vi "Jan25_prot.vi"() -> ()   [LabVIEW 2020]
uses:
  <vilib>/Utility/error.llb/DialogType.ctl
  <vilib>/Analysis/3filter.llb/Filter Passband Type.ctl
  <vilib>/DAQmx/read.llb/DAQmx Read (Analog 1D DBL NChan 1Samp).vi
  <vilib>/DAQmx/create/channels.llb/DAQmx Create Channel (AI-Voltage-Basic).vi
  <vilib>/DAQmx/configure/timing.llb/DAQmx Timing (Sample Clock).vi
  <vilib>/DAQmx/miscellaneous.llb/DAQmx Fill In Error Info.vi
  <vilib>/Analysis/3filter.llb/Butterworth Filter (DBL).vi
  <vilib>/Utility/file.llb/Write Delimited Spreadsheet (string).vi
  <vilib>/Utility/file.llb/Write Delimited Spreadsheet (DBL).vi
  <vilib>/Analysis/NI_AALBase.lvlib
  <vilib>/ptbypt/NI_PtbyPt.lvlib
panel:
  out "Current value":dbl
  in  "Current sin":bool
  in  "Current":dbl
  in  "Sin f (Hz)":dbl
  out "Delay (sec)":dbl
  out "T tot saved":bool
  out "T start saved":bool
  out "Motor":dynamicdata(graph)
  out "T_next":dbl
  out "T_tot":dbl
  in  "Choose Manual Mode":string(combo)
  out "Actual Swing":bool
  out "N° step Max":i32
  in  "Choose Automatic Mode":string(combo)
  in  "START":bool
  out "Step Number":i32
  out "Step Counted":bool
  out "Time to Peak (sec)":dbl=200.0
  out "Swing ON Time (sec)":dbl
  in  "Only pre-tension load":bool
  out "Gyro":dynamicdata(graph)
  out "Max Square Wave duration (sec)":dbl
  out "Swing Start Time (sec)":dbl
  out "Time Saved":bool
  out "Pre-Tension Load (N)":dbl
  out "Target Load (N)":dbl=2.0
  out "Release":bool
  out "Pull":bool
  in  "Working Mode":string(combo)
  out "Load Cell":dbl
  in  "Pull CMD":bool
  in  "Release CMD":bool
  out "Load Cell":dynamicdata(graph)
  in  "Master Stop":bool
  out "Consumer Loop Speed (ms)":u32
  out "Producer Loop Speed (ms)":u32
  out "Swing":bool
  out "Force Plate":dynamicdata(graph)
  out "Accelerometers":dynamicdata(graph)
  out "Enlapsed Time (sec)":dbl
  # "Choose work mode"
  # "Manual"
  # "Automatic"
  # "Ramp Between-Step Mode"
  # "Ramp Within-Step Mode"
  # "Indicators"
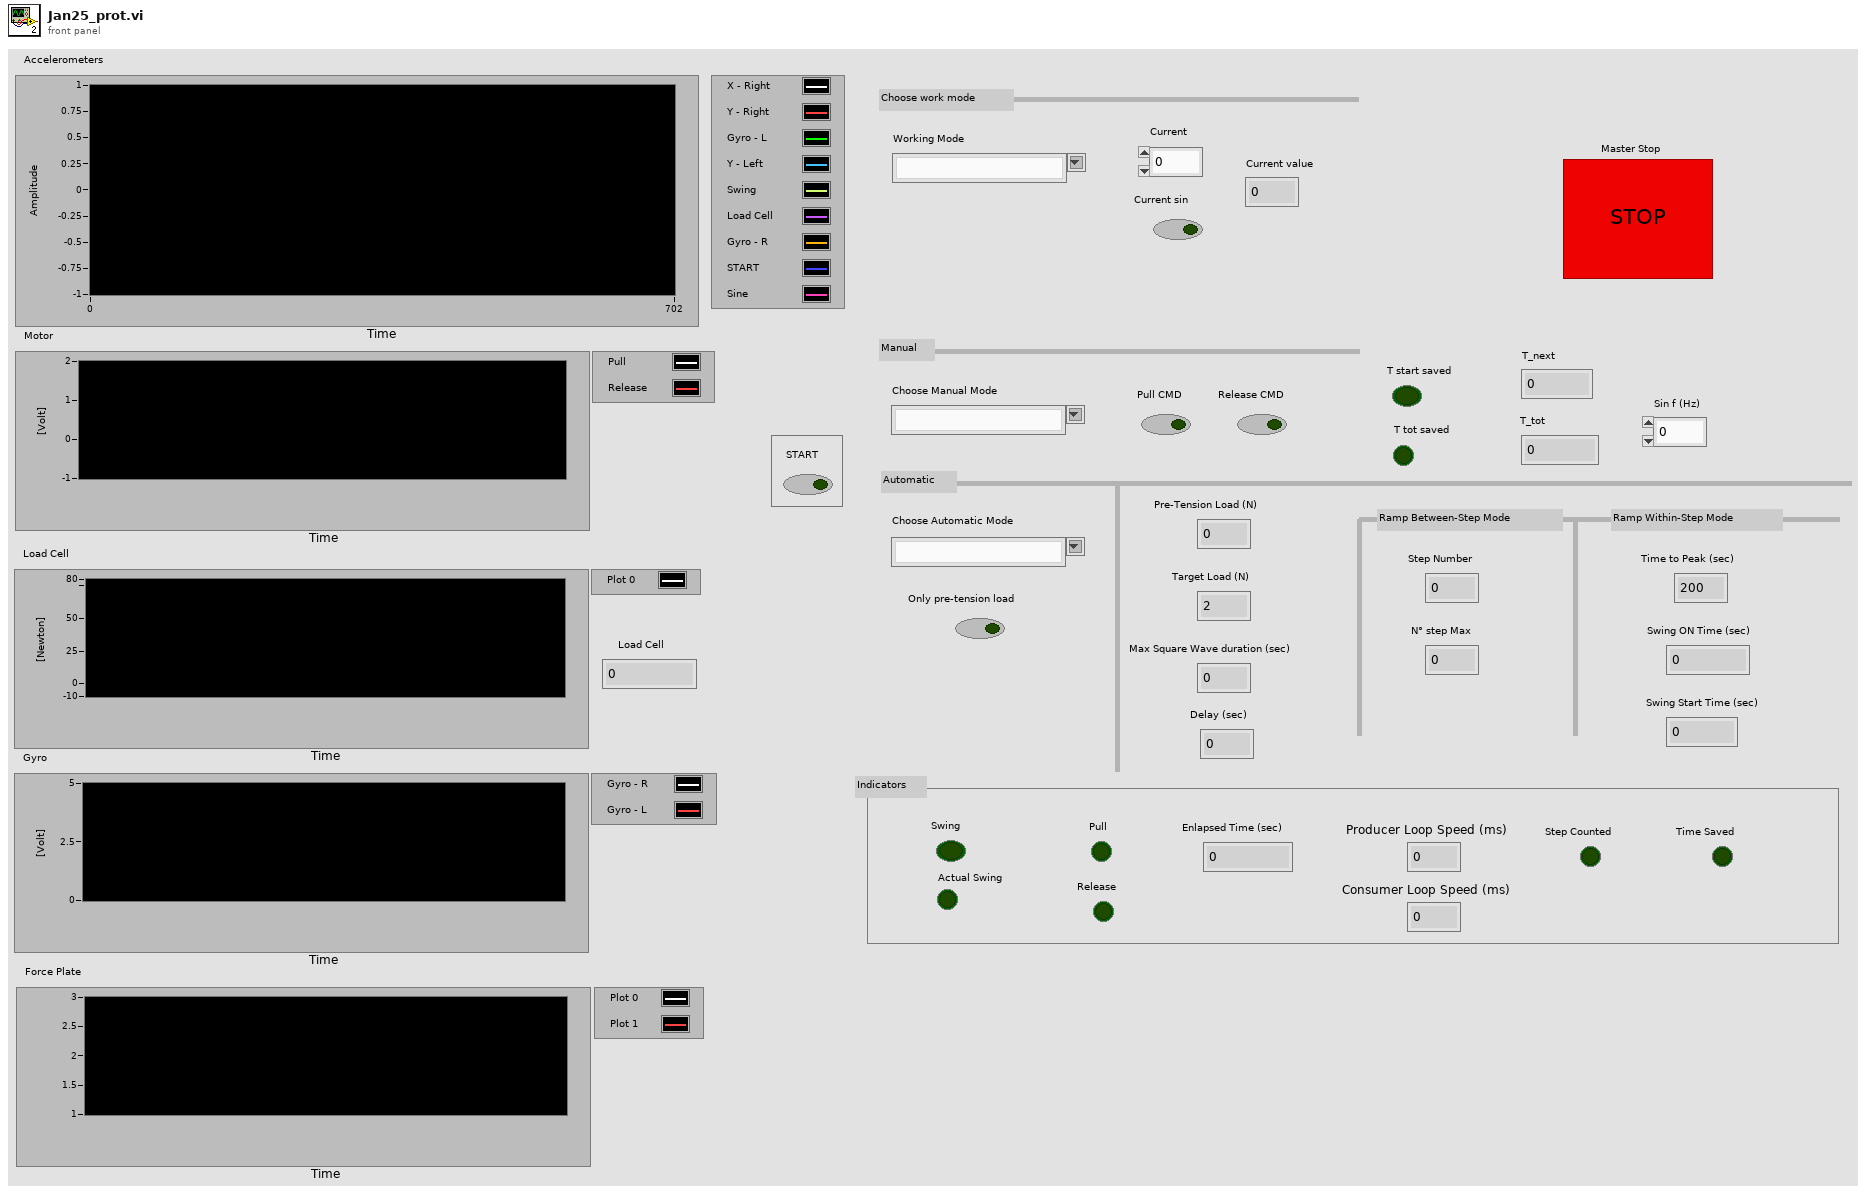
[diagram p1: front panel]
types:
  T1 = typedef "DialogType.ctl" = u16
  T2 = typedef "NI_AALBase.lvlib/Filter Passband Type.ctl" = enum32{"Lowpass", "Highpass", "Bandpass", "Bandstop"}
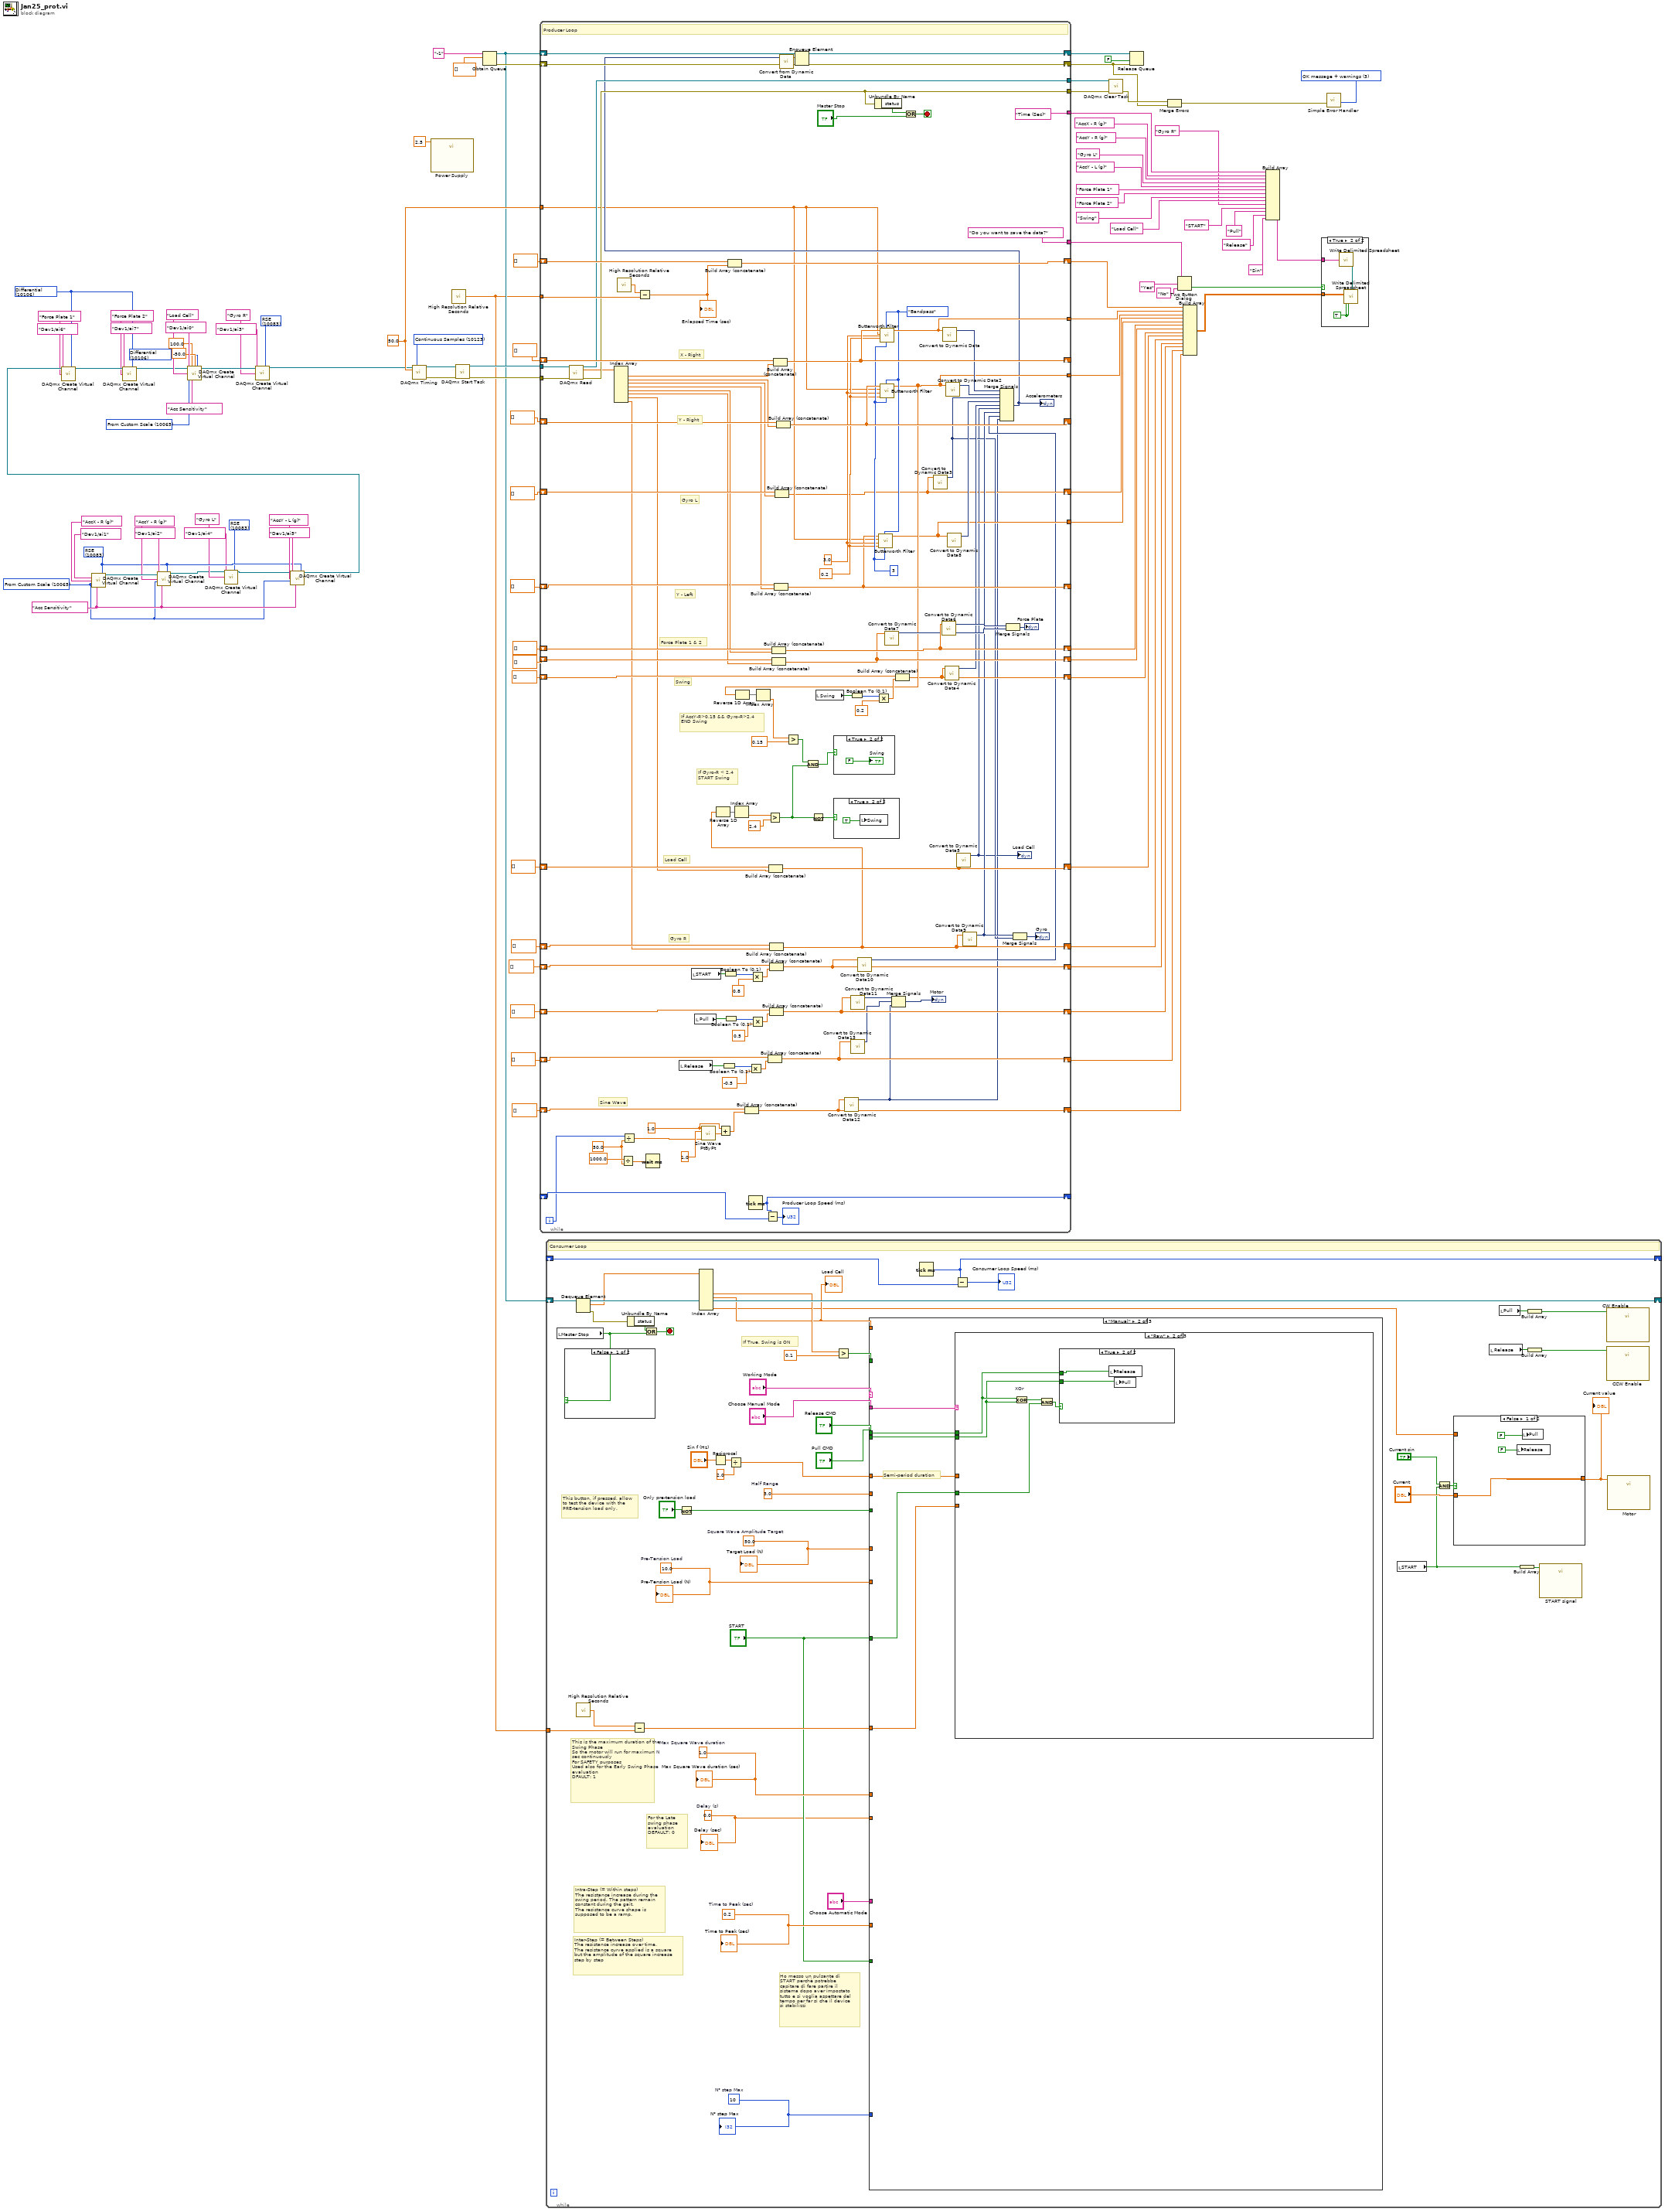
[diagram p0: block diagram]
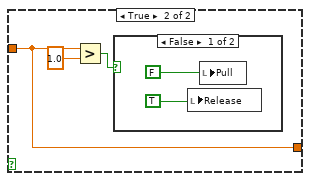
[diagram p2: hidden frame]
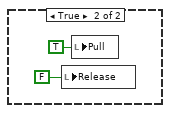
[diagram p3: hidden frame]
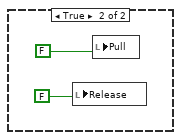
[diagram p4: hidden frame]
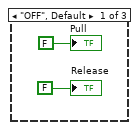
[diagram p5: hidden frame]
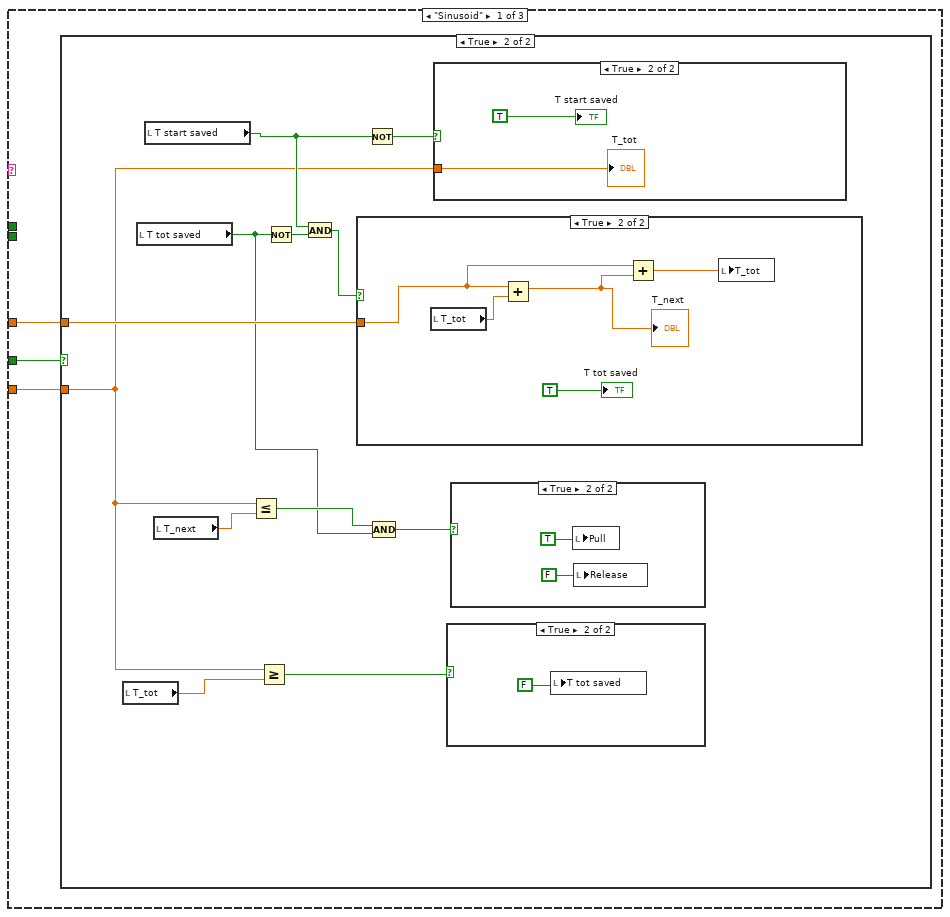
[diagram p6: hidden frame]
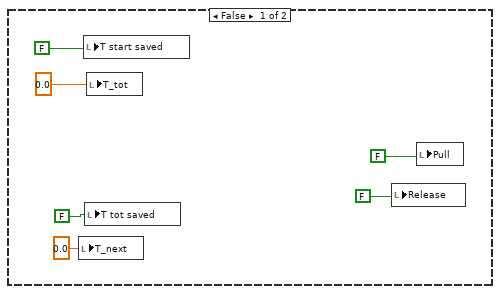
[diagram p7: hidden frame]
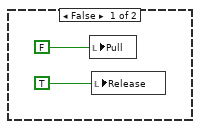
[diagram p10: hidden frame]
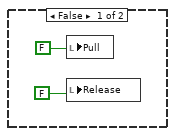
[diagram p12: hidden frame]
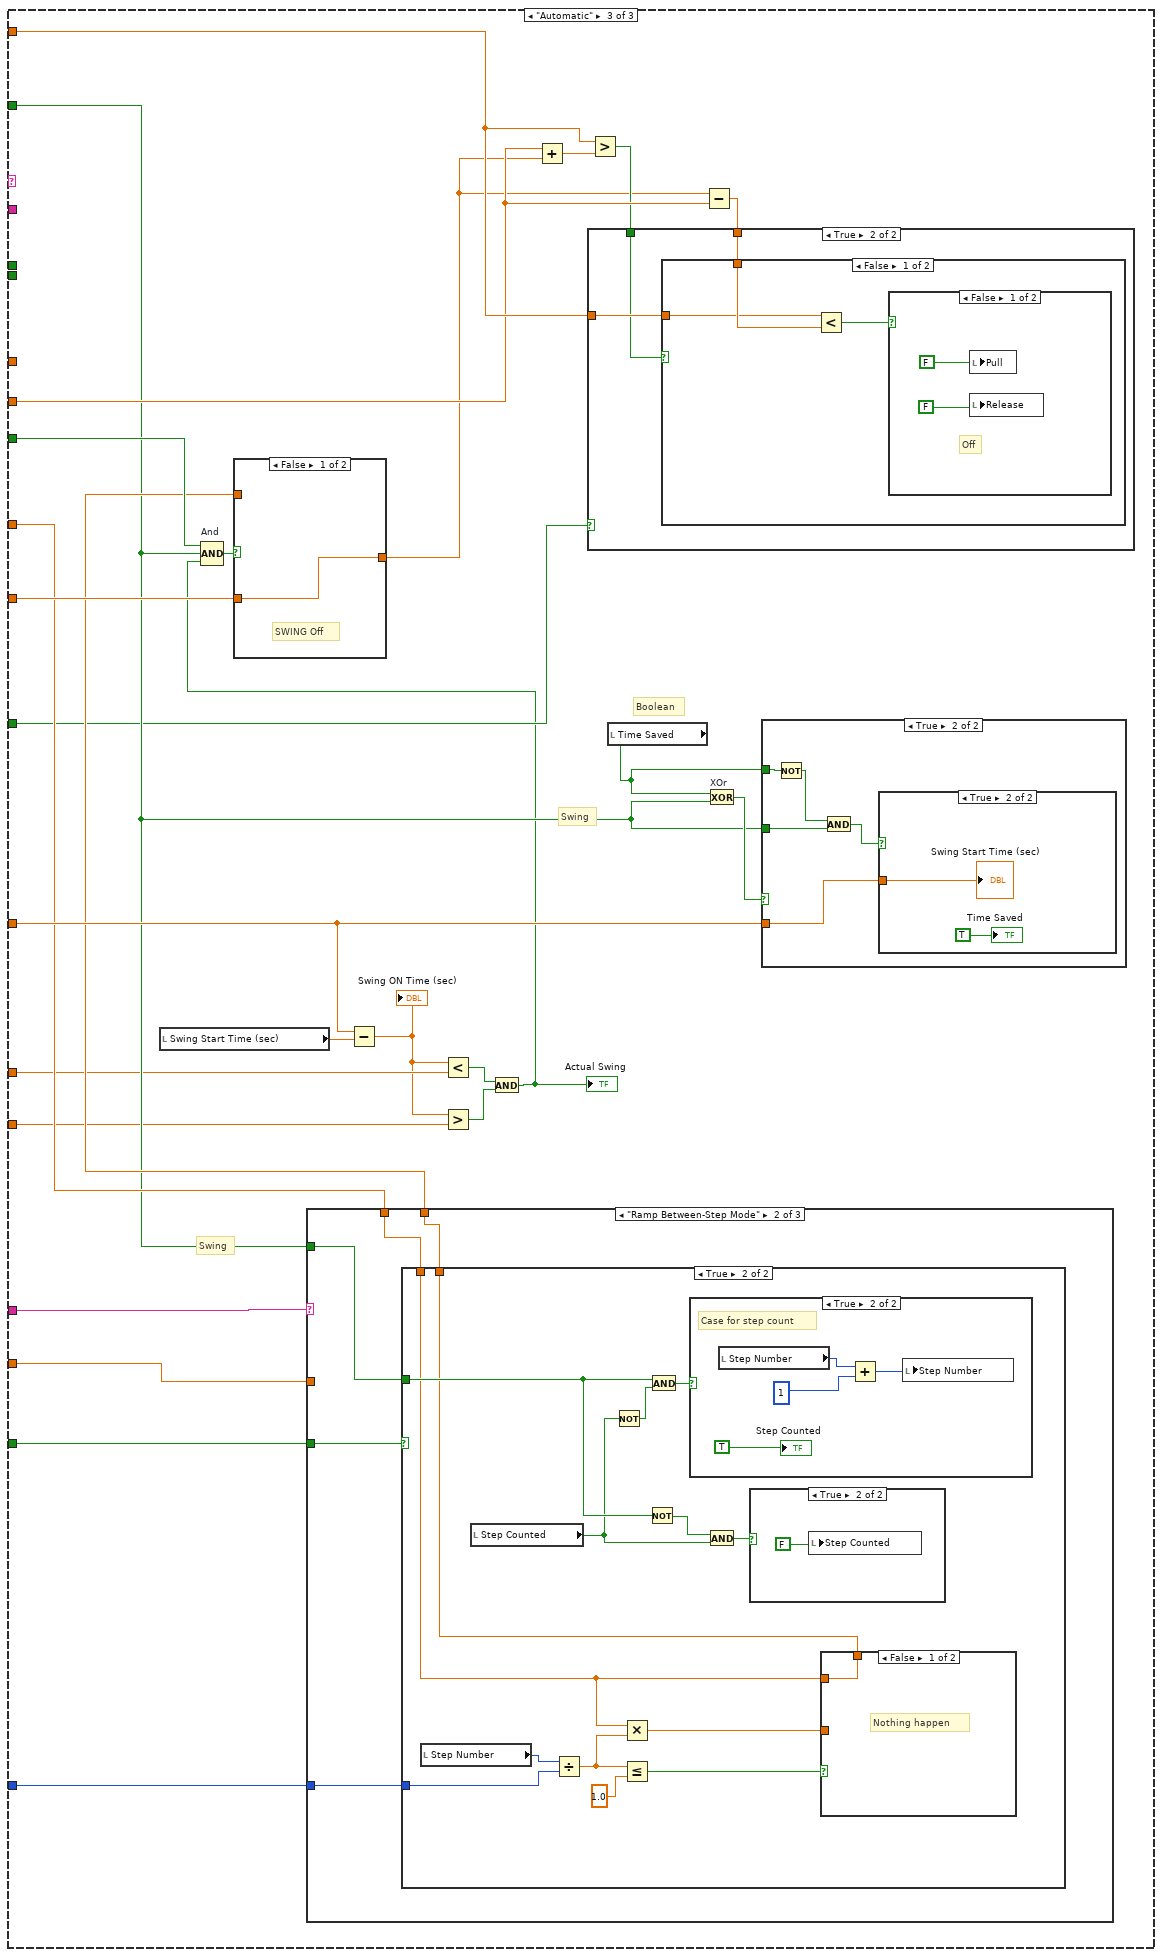
[diagram p14: hidden frame]
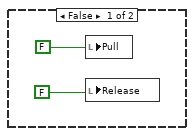
[diagram p15: hidden frame]
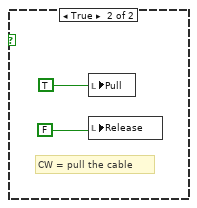
[diagram p16: hidden frame]
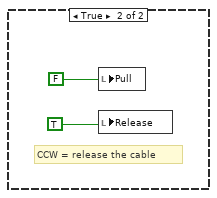
[diagram p17: hidden frame]
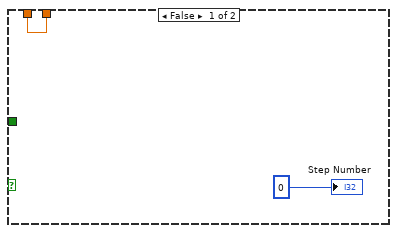
[diagram p19: hidden frame]
diagram:
  w17 = 10083 items=["Default"=-1, "RSE"=10083, "NRSE"=10078, "Differential"=10106, "Pseudodifferential"=12529] ("input terminal configuration")
  w20 = 10106 items=["Default"=-1, "RSE"=10083, "NRSE"=10078, "Differential"=10106, "Pseudodifferential"=12529] ("input terminal configuration")
  w21 = 10083 items=["Default"=-1, "RSE"=10083, "NRSE"=10078, "Differential"=10106, "Pseudodifferential"=12529] ("input terminal configuration")
  w31 = 10065 items=["Volts"=10348, "From Custom Scale"=10065] ("units")
  w46 = T1 3 items=["no dialog", "OK message", "continue or stop message", "OK message + warnings", "continue/stop + warnings"] ("type of dialog (OK msg:1)")
  w36 = 10065 items=["Volts"=10348, "From Custom Scale"=10065] ("units")
  w37 = tag "Acc Sensitivity" ("custom scale name")
  w56 = 10106 items=["Default"=-1, "RSE"=10083, "NRSE"=10078, "Differential"=10106, "Pseudodifferential"=12529] ("input terminal configuration")
  w74 = 10123 items=["Finite Samples"=10178, "Continuous Samples"=10123, "Hardware Timed Single Point"=12522] ("sample mode")
  w69 = 50.0 ("rate")
  w39 = 10083 items=["Default"=-1, "RSE"=10083, "NRSE"=10078, "Differential"=10106, "Pseudodifferential"=12529] ("input terminal configuration")
  n1 = call-poly <vilib>:"DAQmx Create Virtual Channel.vi"("input terminal configuration"=w39, "physical channels"=tag "Dev1/ai1" ("Physical channels"), "name to assign"="AccX - R (g)", "units"=w36, "custom scale name"=w37) -> ("task out"=w68:refnum<k21>)  [unwired: 9 in, 1 out]
  n2 = call-poly <vilib>:"DAQmx Create Virtual Channel.vi"("task in"=w68, "input terminal configuration"=w39, "physical channels"=tag "Dev1/ai2", "name to assign"="AccY - R (g)", "units"=w36, "custom scale name"=w37) -> ("task out"=w16:refnum<k21>)  [unwired: 8 in, 1 out]
  n3 = call-poly <vilib>:"DAQmx Create Virtual Channel.vi"("task in"=w16, "input terminal configuration"=w17, "physical channels"=tag "Dev1/ai4", "name to assign"="Gyro L") -> ("task out"=w15:refnum<k21>)  [unwired: 10 in, 1 out]
  n4 = call-poly <vilib>:"DAQmx Create Virtual Channel.vi"("task in"=w15, "input terminal configuration"=w39, "physical channels"=tag "Dev1/ai5", "name to assign"="AccY - L (g)", "units"=w36, "custom scale name"=w37) -> ("task out"=w67:refnum<k21>)  [unwired: 8 in, 1 out]
  n5 = call-poly <vilib>:"DAQmx Create Virtual Channel.vi"("task in"=w67, "input terminal configuration"=w56, "physical channels"=tag "Dev1/ai6", "name to assign"="Force Plate 1" ("element")) -> ("task out"=w62:refnum<k21>)  [unwired: 10 in, 1 out]
  n6 = call-poly <vilib>:"DAQmx Create Virtual Channel.vi"("task in"=w62, "input terminal configuration"=w56, "physical channels"=tag "Dev1/ai7", "name to assign"="Force Plate 2" ("element")) -> ("task out"=w38:refnum<k21>)  [unwired: 10 in, 1 out]
  n7 = call-poly <vilib>:"DAQmx Create Virtual Channel.vi"("task in"=w38, "maximum value"=100.0, "minimum value"=-50.0, "input terminal configuration"=w20, "physical channels"=tag "Dev1/ai0", "name to assign"="Load Cell", "units"=w31, "custom scale name"=tag "Acc Sensitivity") -> ("task out"=w27:refnum<k21>)  [unwired: 6 in, 1 out]
  n8 = call-poly <vilib>:"DAQmx Create Virtual Channel.vi"("task in"=w27, "input terminal configuration"=w21, "physical channels"=tag "Dev1/ai3", "name to assign"="Gyro R") -> ("task out"=w14:refnum<k21>)  [unwired: 10 in, 1 out]
  n9 = call-poly <vilib>:"DAQmx Timing.vi"("task/channels in"=w14, "sample mode"=w74, "rate"=w69) -> ("task out"=w73:refnum<k21>, "error out"=w72:errorcluster)  [unwired: 11 in]
  n10 = call "Power Supply"("data"=2.5) -> ()  [unwired: 17 in, 2 out]
  n11 = call <vilib>:"High Resolution Relative Seconds.vi"() -> ("relative seconds"=w28:dbl)
  n12 = call <vilib>:"DAQmx Start Task.vi"("task/channels in"=w73, "error in"=w72) -> ("task out"=w71:refnum<k21>, "error out"=w70:errorcluster)  [unwired: 12 in]
  n13 = Obtain Queue(name (unnamed)="-1", element data type=dbl[] []) -> (queue out=w42:refnum<queue>, error out=w51:errorcluster)  [unwired: 3 in, 1 out]
  n14 = while {
    tunnel: w71 -> [w220]
    tunnel: w70 -> [w219]
    tunnel: w28 -> [w217]
    shift-right: [w202] -> w101
    shift-left: dbl[] [] -> [w215]
    shift-right: [w205] -> _
    shift-left: dbl[] [] -> [w214]
    shift-right: [w204] -> _
    shift-left: dbl[] [] -> [w213]
    tunnel: ["Time (Sec)"] -> w77
    tunnel: ["Do you want to save the data?" ("message")] -> w93
    shift-right: [w169] -> w81
    shift-left: dbl[] [] -> [w210]
    shift-right: [w139] -> w13
    shift-left: dbl[] [] -> [w203]
    shift-right: [w193] -> w79
    shift-left: dbl[] [] -> [w196]
    shift-right: [w191] -> w80
    shift-left: dbl[] [] -> [w195]
    tunnel: [w189] -> w83
    tunnel: [w172] -> w82
    shift-right: [w182] -> _
    shift-left: dbl[] [] -> [w181]
    tunnel: [w167] -> w78
    tunnel: w69 -> [w143]
    shift-right: [w174] -> _
    shift-left: _ -> [w173]
    shift-right: [w161] -> w50
    shift-left: w42 -> [w162]
    shift-right: [w159] -> w43
    shift-left: w51 -> [w160]
    tunnel: [w166] -> w48
    tunnel: [w163] -> w47
    shift-right: [w154] -> w34
    shift-left: dbl[] [] -> [w153]
    shift-right: [w148] -> w23
    shift-left: dbl[] [] -> [w151]
    shift-right: [w133] -> w10
    shift-left: dbl[] [] -> [w138]
    shift-right: [w125] -> w8
    shift-left: dbl[] [] -> [w126]
    shift-right: [w105] -> w5
    shift-left: dbl[] [] -> [w121]
    shift-right: [w118] -> w3
    shift-left: dbl[] [] -> [w119]
    i -> [w114]
    stop <- w164 stop-if-true
    w112 = 50.0 ("amplitude")
    w108 = 1.0 ("amplitude")
    w186 = 3 ("order")
    w184 = 0.2 ("low cutoff freq: fl")
    w185 = 3.0 ("high cutoff freq: fh")
    w180 = Filter_Passband_Type."Bandpass" ("filter type")
    # "Sine Wave"
    # "Gyro L"
    # "Gyro R"
    # "X - Right"
    # "Y - Right"
    # "Y - Left"
    # "Force Plate 1 & 2"
    # "Swing"
    # "Load Cell"
    # "If Gyro-R < 2.4\nSTART Swing"
    # "If AccY-R>0.15 && Gyro-R>2.4\nEND Swing"
    # "Producer Loop"
    n15 = call-poly <vilib>:"DAQmx Read.vi"("task/channels in"=w220, "error in"=w219) -> ("task out"=w166:refnum<k21>, "data"=w158:dbl[], "error out"=w163:errorcluster)  [unwired: 11 in]
    n16 = Index Array(array=w158) -> (element #1=w179:dbl, element #2=w178:dbl, element #3=w177:dbl, element #4=w176:dbl, element #5=w187:dbl, element #6=w188:dbl, element #7=w152:dbl, element #8=w150:dbl)  [unwired: 8 in]
    n17 = call <vilib>:"High Resolution Relative Seconds.vi"() -> ("relative seconds"=w218:dbl)
    n18 = Divide(x=1000.0, y=w112) -> (x/y=w111:dbl)
    n19 = Divide(x=w114, y=w112) -> (x/y=w115:dbl)
    n20 = Subtract(x=w218, y=w217) -> (x-y=w216:dbl)
    "Enlapsed Time (sec)" <- w216
    n21 = Wait (ms)(milliseconds to wait=w111) -> ()  [unwired: 1 out]
    n22 = local read "Release"() -> (w117:bool)
    n23 = local read "START"() -> (w134:bool)
    n24 = local read "Pull"() -> (w127:bool)
    n25 = call <vilib>:"Sine Wave PtByPt.vi"("time"=w115, "frequency"=1.0, "amplitude"=w108) -> ("sine wave"=w110:dbl)  [unwired: 1 in]
    n26 = Add(x=w108, y=w110) -> (x+y=w109:dbl)
    n27 = Boolean To (0,1)(Boolean=w117) -> (0, 1=w123:i16)
    n28 = Boolean To (0,1)(Boolean=w134) -> (0, 1=w137:i16)
    n29 = Boolean To (0,1)(Boolean=w127) -> (0, 1=w129:i16)
    n30 = Build Array (concatenate)(w215, w216) -> (w202:dbl[])
    n31 = Build Array (concatenate)(w119, w109) -> (w118:dbl[])
    n32 = Tick Count (ms)() -> (millisecond timer value=w174:u32)
    n33 = Multiply(x=w123, y=-0.5) -> (x*y=w124:dbl)
    n34 = Multiply(x=w137, y=0.8) -> (x*y=w135:dbl)
    n35 = Multiply(x=w129, y=0.5) -> (x*y=w130:dbl)
    n36 = Subtract(x=w174, y=w173) -> (x-y=→"Producer Loop Speed (ms)":u32)
    n37 = Build Array (concatenate)(w121, w124) -> (w105:dbl[])
    n38 = Build Array (concatenate)(w153, w152) -> (w154:dbl[])
    n39 = Build Array (concatenate)(w151, w150) -> (w148:dbl[])
    n40 = Reverse 1D Array(array=w148) -> (reversed array=w198:dbl[])
    n41 = Index Array(array=w198) -> (element=w197:dbl)  [unwired: 1 in]
    n42 = Greater?(x=w197, y=2.4) -> (0:w144:bool)
    n43 = Build Array (concatenate)(w138, w135) -> (w133:dbl[])
    n44 = Build Array (concatenate)(w126, w130) -> (w125:dbl[])
    n45 = Build Array (concatenate)(w196, w187) -> (w193:dbl[])
    n46 = Build Array (concatenate)(w195, w188) -> (w191:dbl[])
    n47 = Build Array (concatenate)(w214, w179) -> (w205:dbl[])
    n48 = Build Array (concatenate)(w181, w176) -> (w182:dbl[])
    n49 = Build Array (concatenate)(w203, w177) -> (w139:dbl[])
    n50 = Build Array (concatenate)(w213, w178) -> (w204:dbl[])
    n51 = Not(x=w144) -> (.not. x?=w145:bool)
    n52 = local read "Swing"() -> (w131:bool)
    n53 = case shown="True" w145 {
      frame False {
      }
      frame True {
        n54 = local write "Swing"(TRUE) -> ()
      }
    }
    n55 = call "Convert to Dynamic Data12"("Array"=w118) -> ("Dynamic Data Type"=w104:dynamicdata)  [unwired: 3 in]
    n56 = Boolean To (0,1)(Boolean=w131) -> (0, 1=w208:i16)
    n57 = call "Convert to Dynamic Data11"("Array"=w125) -> ("Dynamic Data Type"=w120:dynamicdata)  [unwired: 3 in]
    n58 = call "Convert to Dynamic Data13"("Array"=w105) -> ("Dynamic Data Type"=w106:dynamicdata)  [unwired: 3 in]
    n59 = call "Convert to Dynamic Data10"("Array"=w133) -> ("Dynamic Data Type"=w132:dynamicdata)  [unwired: 3 in]
    n60 = Unbundle By Name(w163) -> ("status"=w165:bool)
    n61 = Multiply(x=w208, y=0.2) -> (x*y=w209:dbl)
    n62 = call-poly <vilib>:"Butterworth Filter.vi"("order"=w186, "filter type"=w180, "low cutoff freq: fl"=w184, "high cutoff freq: fh"=w185, "sampling freq: fs"=w143, "X"=w182) -> ("Filtered X"=w167:dbl[])  [unwired: 2 in, 1 out]
    n63 = call-poly <vilib>:"Butterworth Filter.vi"("order"=w186, "filter type"=w180, "low cutoff freq: fl"=w184, "high cutoff freq: fh"=w185, "sampling freq: fs"=w143, "X"=w205) -> ("Filtered X"=w189:dbl[])  [unwired: 2 in, 1 out]
    n64 = call-poly <vilib>:"Butterworth Filter.vi"("order"=w186, "filter type"=w180, "low cutoff freq: fl"=w184, "high cutoff freq: fh"=w185, "sampling freq: fs"=w143, "X"=w204) -> ("Filtered X"=w172:dbl[])  [unwired: 2 in, 1 out]
    n65 = Reverse 1D Array(array=w172) -> (reversed array=w206:dbl[])
    n66 = Index Array(array=w206) -> (element=w171:dbl)  [unwired: 1 in]
    n67 = Greater?(x=w171, y=0.15) -> (0:w146:bool)
    n68 = And(x=w146, y=w144) -> (x .and. y?=w147:bool)
    n69 = case shown="True" w147 {
      frame False {
      }
      frame True {
        "Swing" <- FALSE
      }
    }
    n70 = call "Convert to Dynamic Data7"("Array"=w191) -> ("Dynamic Data Type"=w190:dynamicdata)  [unwired: 3 in]
    n71 = Merge Signals(w120, w106, w104) -> (→"Motor":dynamicdata)
    n72 = Build Array (concatenate)(w210, w209) -> (w169:dbl[])
    n73 = Or(x=w165, y="Master Stop") -> (x .or. y?=w164:bool)
    n74 = call "Convert to Dynamic Data3"("Array"=w139) -> ("Dynamic Data Type"=w141:dynamicdata)  [unwired: 3 in]
    n75 = call "Convert to Dynamic Data6"("Array"=w193) -> ("Dynamic Data Type"=w192:dynamicdata)  [unwired: 3 in]
    n76 = call "Convert to Dynamic Data"("Array"=w189) -> ("Dynamic Data Type"=w201:dynamicdata)  [unwired: 3 in]
    n77 = call "Convert to Dynamic Data4"("Array"=w169) -> ("Dynamic Data Type"=w168:dynamicdata)  [unwired: 3 in]
    n78 = call "Convert to Dynamic Data2"("Array"=w172) -> ("Dynamic Data Type"=w200:dynamicdata)  [unwired: 3 in]
    n79 = call "Convert to Dynamic Data8"("Array"=w167) -> ("Dynamic Data Type"=w183:dynamicdata)  [unwired: 3 in]
    n80 = call "Convert to Dynamic Data5"("Array"=w154) -> ("Dynamic Data Type"=w140:dynamicdata)  [unwired: 3 in]
    "Load Cell" <- w140
    n81 = call "Convert to Dynamic Data9"("Array"=w148) -> ("Dynamic Data Type"=w149:dynamicdata)  [unwired: 3 in]
    n82 = Merge Signals(w201, w200, w141, w183, w168, w140, w149, w132, w104) -> (w156:dynamicdata)
    "Accelerometers" <- w156
    n83 = call "Convert from Dynamic Data"("Dynamic Data Type"=w156) -> ("Array"=w155:dbl[])  [unwired: 3 in]
    n84 = Enqueue Element(queue=w162, element=w155, error in (no error)=w160) -> (queue out=w161:refnum<queue>, error out=w159:errorcluster)  [unwired: 1 in, 1 out]
    n85 = Merge Signals(w192, w190) -> (→"Force Plate":dynamicdata)
    n86 = Merge Signals(w149, w141) -> (→"Gyro":dynamicdata)
  }
  n87 = while {
    shift-right: [w268] -> _
    shift-left: w42 -> [w269]
    shift-right: [w265] -> _
    shift-left: _ -> [w266]
    tunnel: w28 -> [w244]
    stop <- w263 stop-if-true
    w232 = 0.0  # Delay (s)
    w237 = 10  # N° step Max
    w239 = 0.2  # Time to Peak (sec)
    w242 = 1.0  # Max Square Wave duration
    w246 = 3.0  # Half Range
    w247 = 10.0  # Pre-Tension Load
    w248 = 50.0  # Square Wave Amplitude Target
    # "For the Late swing phase evaluation\nDEFAULT: 0"
    # "This is the maximum duration of the Swing Phase\nSo the motor will run for maximun N sec continuously\nFor SAFETY purposes\nUsed also for the Early Swing Phase evaluation\nDFAULT: 1"
    # "Ho messo un pulsante di \nSTART perchè potrebbe\ncapitare di fare partire il \nsistema dopo aver impostato \ntutto e si voglia aspettare del \ntempo per far si che il device\nsi stabilizzi"
    # "Inter-Step (= Between Steps)\nThe resistance increase over time.\nThe resistance curve applied is a square\nbut the amplitude of the square increase \nstep by step"
    # "Intra-Step (= Within steps) \nThe resistance increase during the\nswing period. The pattern remain \nconstant during the gait.\nThe resistance curve shape is \nsupposed to be a ramp."
    # "This button, if pressed, allow\nto test the device with the\nPRE-tension load only."
    # "If True, Swing is ON"
    # "Consumer Loop"
    n88 = local read "Master Stop"() -> (w249:bool)
    n89 = case shown="False" w249 {
      frame False {
      }
      frame True {
        n90 = local write "Release"(FALSE) -> ()
        n91 = local write "Pull"(FALSE) -> ()
      }
    }
    n92 = Dequeue Element(queue=w269) -> (queue out=w268:refnum<queue>, element=w261:dbl[], error out=w262:errorcluster)  [unwired: 2 in, 1 out]
    n93 = call <vilib>:"High Resolution Relative Seconds.vi"() -> ("relative seconds"=w245:dbl)
    n94 = Unbundle By Name(w262) -> ("status"=w264:bool)
    n95 = Subtract(x=w245, y=w244) -> (x-y=w243:dbl)
    n96 = Or(x=w264, y=w249) -> (x .or. y?=w263:bool)
    n97 = Not(x="Only pre-tension load") -> (.not. x?=w240:bool)
    n98 = Index Array(array=w261) -> (element #5=w260:dbl, element #6=w258:dbl, element #9=w226:dbl)  [unwired: 9 in, 6 out]
    "Load Cell" <- w258
    n99 = Reciprocal(x="Sin f (Hz)") -> (1/x=w231:dbl)
    n100 = Divide(x=w231, y=2.0) -> (x/y=w229:dbl)
    n101 = Greater?(x=w260, y=0.1) -> (0:w250:bool)
    n102 = case shown="\"Manual\"" "Working Mode" {
      tunnel: w258 -> [_ _ w358]
      tunnel: "Release CMD" -> [_ w289 _]
      tunnel: "Pull CMD" -> [_ w288 _]
      tunnel: w250 -> [_ _ w341]
      tunnel: w248 -> [_ _ w346]
      tunnel: w247 -> [_ _ w353]
      tunnel: w246 -> [_ _ w357]
      tunnel: w243 -> [_ w286 w348]
      tunnel: w242 -> [_ _ w337]
      tunnel: w240 -> [_ _ w349]
      tunnel: w239 -> [_ _ w344]
      tunnel: "START" -> [_ _ w340]
      tunnel: "Choose Automatic Mode" -> [_ _ w342]
      tunnel: w237 -> [_ _ w339]
      tunnel: "START" -> [_ w285 w338]
      tunnel: "Choose Manual Mode" -> [_ w287 _]
      tunnel: w229 -> [_ w284 _]
      tunnel: w232 -> [_ _ w336]
      frame "OFF", Default {
        "Pull" <- FALSE
        "Release" <- FALSE
      }
      frame "Manual" {
        # "Semi-period duration"
        n103 = case shown="\"Raw\"" w287 {
          tunnel: w289 -> [_ w327 _]
          tunnel: w288 -> [_ w326 _]
          tunnel: w286 -> [w291 _ _]
          tunnel: w285 -> [w292 w323 _]
          tunnel: w284 -> [w290 _ _]
          frame "Sinusoid" {
            n104 = case shown="True" w292 {
              tunnel: w291 -> [_ w301]
              tunnel: w290 -> [_ w304]
              frame False {
                n105 = local write "T_next"(0.0 ("T_next")) -> ()
                n106 = local write "T start saved"(FALSE) -> ()
                n107 = local write "T tot saved"(FALSE) -> ()
                n108 = local write "T_tot"(0.0 ("Sin Start")) -> ()
                n109 = local write "Release"(FALSE) -> ()
                n110 = local write "Pull"(FALSE) -> ()
              }
              frame True {
                n111 = local read "T_tot"() -> (w300:dbl)
                n112 = local read "T tot saved"() -> (w302:bool)
                n113 = local read "T start saved"() -> (w308:bool)
                n114 = local read "T_next"() -> (w305:dbl)
                n115 = Less Or Equal?(x=w301, y=w305) -> (x <= y?=w306:bool)
                n116 = Greater Or Equal?(x=w301, y=w300) -> (x >= y?=w299:bool)
                n117 = Not(x=w302) -> (.not. x?=w307:bool)
                n118 = And(x=w308, y=w307) -> (x .and. y?=w303:bool)
                n119 = case shown="True" w303 {
                  tunnel: w304 -> [_ w314]
                  frame False {
                  }
                  frame True {
                    n120 = local read "T_tot"() -> (w316:dbl)
                    n121 = Add(x=w314, y=w316) -> (x+y=w312:dbl)
                    "T_next" <- w312
                    n122 = Add(x=w314, y=w312) -> (x+y=w313:dbl)
                    n123 = local write "T_tot"(w313) -> ()
                    "T tot saved" <- TRUE
                  }
                }
                n124 = Not(x=w308) -> (.not. x?=w310:bool)
                n125 = Compound Arithmetic op=AND(w306, w302) -> (w309:bool)
                n126 = case shown="True" w310 {
                  tunnel: w301 -> [_ w322]
                  frame False {
                  }
                  frame True {
                    "T_tot" <- w322
                    "T start saved" <- TRUE
                  }
                }
                n127 = case shown="True" w299 {
                  frame False {
                  }
                  frame True {
                    n128 = local write "T tot saved"(FALSE) -> ()
                  }
                }
                n129 = case shown="True" w309 {
                  frame False {
                    n130 = local write "Pull"(FALSE) -> ()
                    n131 = local write "Release"(TRUE) -> ()
                  }
                  frame True {
                    n132 = local write "Pull"(TRUE) -> ()
                    n133 = local write "Release"(FALSE) -> ()
                  }
                }
              }
            }
          }
          frame "Raw" {
            n134 = Exclusive Or "XOr"(1:w326, 2:w327) -> (0:w324:bool)
            n135 = And(x=w324, y=w323) -> (x .and. y?=w325:bool)
            n136 = case shown="True" w325 {
              tunnel: w327 -> [_ w330]
              tunnel: w326 -> [_ w331]
              frame False {
                n137 = local write "Pull"(FALSE) -> ()
                n138 = local write "Release"(FALSE) -> ()
              }
              frame True {
                n139 = local write "Release"(w330) -> ()
                n140 = local write "Pull"(w331) -> ()
              }
            }
          }
          frame "OFF", Default {
          }
        }
      }
      frame "Automatic" {
        # "Swing"
        # "Boolean"
        # "Swing"
        n141 = local read "Swing Start Time (sec)"() -> (w347:dbl)
        n142 = case shown="\"Ramp Between-Step Mode\"" w342 {
          tunnel: w346 -> [w373 w376 w403]
          tunnel: [w373 w375 w404] -> w345
          tunnel: w344 -> [_ _ w405]
          tunnel: w341 -> [_ w378 _]
          tunnel: w340 -> [_ w377 w402]
          tunnel: w339 -> [_ w374 _]
          frame "No Ramp", Default {
            # "If the ramp mode is OFF, \nnothing happen. \nThe SWA target remain the same."
          }
          frame "Ramp Between-Step Mode" {
            n143 = case shown="True" w377 {
              tunnel: w378 -> [_ w393]
              tunnel: w376 -> [w379 w382]
              tunnel: [w379 w384] -> w375
              tunnel: w374 -> [_ w387]
              frame False {
                "Step Number" <- 0
              }
              frame True {
                n144 = local read "Step Number"() -> (w388:i32)
                n145 = local read "Step Counted"() -> (w391:bool)
                n146 = Divide(x=w388, y=w387) -> (x/y=w383:dbl)
                n147 = Not(x=w391) -> (.not. x?=w392:bool)
                n148 = Multiply(x=w382, y=w383) -> (x*y=w381:dbl)
                n149 = Less Or Equal?(x=w383, y=1.0) -> (x <= y?=w385:bool)
                n150 = Not(x=w393) -> (.not. x?=w389:bool)
                n151 = And(x=w393, y=w392) -> (x .and. y?=w394:bool)
                n152 = case shown="True" w394 {
                  frame False {
                  }
                  frame True {
                    # "Case for step count"
                    n153 = local read "Step Number"() -> (w400:i32)
                    n154 = Add(x=w400, y=1) -> (x+y=w399:i32)
                    n155 = local write "Step Number"(w399) -> ()
                    "Step Counted" <- TRUE
                  }
                }
                n156 = And(x=w389, y=w391) -> (x .and. y?=w390:bool)
                n157 = case shown="True" w390 {
                  frame False {
                  }
                  frame True {
                    n158 = local write "Step Counted"(FALSE) -> ()
                  }
                }
                n159 = case shown="False" w385 {
                  tunnel: w382 -> [w395 _]
                  tunnel: [w395 w396] -> w384
                  tunnel: w381 -> [_ w396]
                  frame False {
                    # "Nothing happen"
                  }
                  frame True {
                  }
                }
              }
            }
          }
          frame "Ramp Within-Step Mode" {
            n160 = case shown="True" w402 {
              tunnel: w405 -> [_ w413]
              tunnel: [w406 w411] -> w404
              tunnel: w403 -> [w406 w407]
              frame False {
              }
              frame True {
                n161 = local read "Swing ON Time (sec)"() -> (w414:dbl)
                n162 = Divide(x=w414, y=w413) -> (x/y=w409:dbl)
                n163 = Less Or Equal?(x=w409, y=1.0) -> (x <= y?=w408:bool)
                n164 = Multiply(x=w407, y=w409) -> (x*y=w412:dbl)
                n165 = case shown="False" w408 {
                  tunnel: w412 -> [_ w416]
                  tunnel: [w415 w416] -> w411
                  tunnel: w407 -> [w415 _]
                  frame False {
                    # "Nothing Happen"
                  }
                  frame True {
                  }
                }
              }
            }
          }
        }
        n166 = Subtract(x=w348, y=w347) -> (x-y=w335:dbl)
        "Swing ON Time (sec)" <- w335
        n167 = Less?(x=w335, y=w337) -> (x < y?=w333:bool)
        n168 = Greater?(x=w335, y=w336) -> (0:w334:bool)
        n169 = And(x=w333, y=w334) -> (x .and. y?=w332:bool)
        "Actual Swing" <- w332
        n170 = Compound Arithmetic op=AND "And"(w349, w341, w332) -> (w343:bool)
        n171 = case shown="False" w343 {
          tunnel: w345 -> [_ w426]
          tunnel: w353 -> [w425 _]
          tunnel: [w425 w426] -> w352
          frame False {
            # "SWING Off"
          }
          frame True {
            # "SWING ON"
          }
        }
        n172 = Add(x=w357, y=w352) -> (x+y=w355:dbl)
        n173 = Greater?(x=w358, y=w355) -> (0:w356:bool)
        n174 = local read "Time Saved"() -> (w350:bool)
        n175 = Subtract(x=w352, y=w357) -> (x-y=w354:dbl)
        n176 = case shown="True" w338 {
          tunnel: w358 -> [_ w363]
          tunnel: w356 -> [_ w362]
          tunnel: w354 -> [_ w361]
          frame False {
            n177 = local write "Pull"(FALSE) -> ()
            n178 = local write "Release"(FALSE) -> ()
          }
          frame True {
            n179 = case shown="False" w362 {
              tunnel: w363 -> [w365 _]
              tunnel: w361 -> [w366 _]
              frame False {
                n180 = Less?(x=w365, y=w366) -> (x < y?=w364:bool)
                n181 = case shown="False" w364 {
                  frame False {
                    # "Off"
                    n182 = local write "Pull"(FALSE) -> ()
                    n183 = local write "Release"(FALSE) -> ()
                  }
                  frame True {
                    # "CW = pull the cable"
                    n184 = local write "Pull"(TRUE) -> ()
                    n185 = local write "Release"(FALSE) -> ()
                  }
                }
              }
              frame True {
                # "CCW = release the cable"
                n186 = local write "Pull"(FALSE) -> ()
                n187 = local write "Release"(TRUE) -> ()
              }
            }
          }
        }
        n188 = Exclusive Or "XOr"(1:w341, 2:w350) -> (0:w351:bool)
        n189 = case shown="True" w351 {
          tunnel: w348 -> [_ w421]
          tunnel: w350 -> [_ w417]
          tunnel: w341 -> [_ w419]
          frame False {
          }
          frame True {
            n190 = Not(x=w417) -> (.not. x?=w418:bool)
            n191 = And(x=w418, y=w419) -> (x .and. y?=w420:bool)
            n192 = case shown="True" w420 {
              tunnel: w421 -> [_ w424]
              frame False {
                n193 = local write "Time Saved"(FALSE) -> ()
              }
              frame True {
                "Swing Start Time (sec)" <- w424
                "Time Saved" <- TRUE
              }
            }
          }
        }
      }
    }
    n194 = Tick Count (ms)() -> (millisecond timer value=w265:u32)
    n195 = Subtract(x=w265, y=w266) -> (x-y=→"Consumer Loop Speed (ms)":u32)
    n196 = local read "START"() -> (w223:bool)
    n197 = And(x="Current sin", y=w223) -> (x .and. y?=w225:bool)
    n198 = case shown="False" w225 {
      tunnel: w226 -> [_ w274]
      tunnel: [w272 w274] -> w228
      tunnel: "Current" -> [w272 _]
      frame False {
        n199 = local write "Release"(FALSE) -> ()
        n200 = local write "Pull"(FALSE) -> ()
      }
      frame True {
        n201 = Greater?(x=w274, y=1.0) -> (0:w273:bool)
        n202 = case shown="False" w273 {
          frame False {
            n203 = local write "Release"(TRUE) -> ()
            n204 = local write "Pull"(FALSE) -> ()
          }
          frame True {
            n205 = local write "Release"(FALSE) -> ()
            n206 = local write "Pull"(TRUE) -> ()
          }
        }
      }
    }
    "Current value" <- w228
    n207 = local read "Release"() -> (w253:bool)
    n208 = local read "Pull"() -> (w254:bool)
    n209 = Build Array(w223) -> (w235:bool[])
    n210 = Build Array(w253) -> (w255:bool[])
    n211 = Build Array(w254) -> (w256:bool[])
    n212 = call "START signal"("data"=w235) -> ()  [unwired: 17 in, 2 out]
    n213 = call "CW Enable"("data"=w256) -> ()  [unwired: 17 in, 2 out]
    n214 = call "CCW Enable"("data"=w255) -> ()  [unwired: 17 in, 2 out]
    n215 = call "Motor"("data"=w228) -> ()  [unwired: 17 in, 2 out]
    "Target Load (N)" <- w248
    "Pre-Tension Load (N)" <- w247
    "Max Square Wave duration (sec)" <- w242
    "Time to Peak (sec)" <- w239
    "N° step Max" <- w237
    "Delay (sec)" <- w232
  }
  n216 = call <vilib>:"DAQmx Clear Task.vi"("task in"=w48, "error in"=w47) -> ("error out"=w44:errorcluster)  [unwired: 13 out]
  n217 = Release Queue(queue=w50, force destroy? (F)=FALSE, error in (no error)=w43) -> ()  [unwired: 3 out]
  n218 = Merge Errors(w44, w43) -> (w45:errorcluster)
  n219 = Two Button Dialog(message=w93, 1:"No" ("F button name (\"Cancel\")"), 2:"Yes" ("T button name (\"OK\")")) -> (T button?=w96:bool)
  n220 = Build Array(w101, w83, w82, w13, w78, w79, w80, w81, w34, w23, w10, w8, w5, w3) -> (w100:dbl[][])
  n221 = Build Array(w77, "AccX - R (g)", "AccY - R (g)", "Gyro L", "AccY - L (g)", "Force Plate 1" ("element"), "Force Plate 2" ("element"), "Swing" ("element"), "Load Cell" ("element"), "Gyro R" ("element"), "START" ("element"), "Pull" ("element"), "Release" ("element"), "Sin" ("element")) -> (w99:string[])
  n222 = case shown="True" w96 {
    tunnel: w100 -> [_ w430]
    tunnel: w99 -> [_ w429]
    frame False {
    }
    frame True {
      w428 = TRUE ("transpose? (no:F)")
      n223 = call-poly <vilib>:"Write Delimited Spreadsheet.vi"("1D data"=w429) -> ("new file path (Not A Path if cancelled)"=w427:path)  [unwired: 13 in, 1 out]
      n224 = call-poly <vilib>:"Write Delimited Spreadsheet.vi"("file path (dialog if empty)"=w427, "2D data"=w430, "append to file? (new file:F)"=w428, "transpose? (no:F)"=w428) -> ()  [unwired: 10 in, 2 out]
    }
  }
  n225 = call <vilib>:"Simple Error Handler.vi"("type of dialog (OK msg:1)"=w46, "error in (no error)"=w45) -> ()  [unwired: 8 out]
